vi "solar_type Script to Messages.vi"(6 "Array Delimiters (1D,2D)":string[](array[string]), 8 "error in (no error)":errorcluster, 11 "Script String":string) -> (0 "error out":errorcluster, 2 "Messages":cluster{"MSG":string, "DATA":variant}[](array[cluster]), 3 "Target":string[](array[string]), 5 "Type":enum8{"CMD", "TLM"}[](array[ring]))   [LabVIEW 2018]
doc: "This converts a SOLAR script string to one or more variant messages. Formatted as:\n<b>CMD|TLM.TARGET:PACKET{\nTYPE:VALUE,\nTYPE:'VALUE',\nTYPE|ENUM0|ENUM1|...:VALUE,\nTYPE_1D:'1,2,3',\nTYPE_2D:'1,2,3;4,5,6'}</b>\n\n<b>TYPE</b>= I8, I16, I32, I64, U8, U16, U32, U64, U8_ENUM, U16_ENUM, U32_ENUM, SGL, DBL, BOOL, STR, PATH, TIME\nTYPE_1D: 1D array (comma ',' delimited) Ex: DBL_1D:'1.23,4.567,8.92'\nTYPE_2D: 2D array (comma ',' & semicolon ';' delimited) Ex: I32_2D:'1,2,3;4,5,6'\nTYPE_ENUM: Enum with type items (pipe '|' delimited) Ex: U16_ENUM|Item 1|Item 2|Item 3:'Item 2'\n\nMyTarget:MyCMD{\nI32:-1234,\nSTR:'Hello World',\nU16_ENUM|Item1|Item2|Item3:'Item2',\nBOOL:true,\nTIME:'yyyy-mm-dd_hh:mm:ss.uuuuuu',\nPATH:'C:\\Data\\test.txt',\nU8_2D:'1,2,3;4,5,6'}"
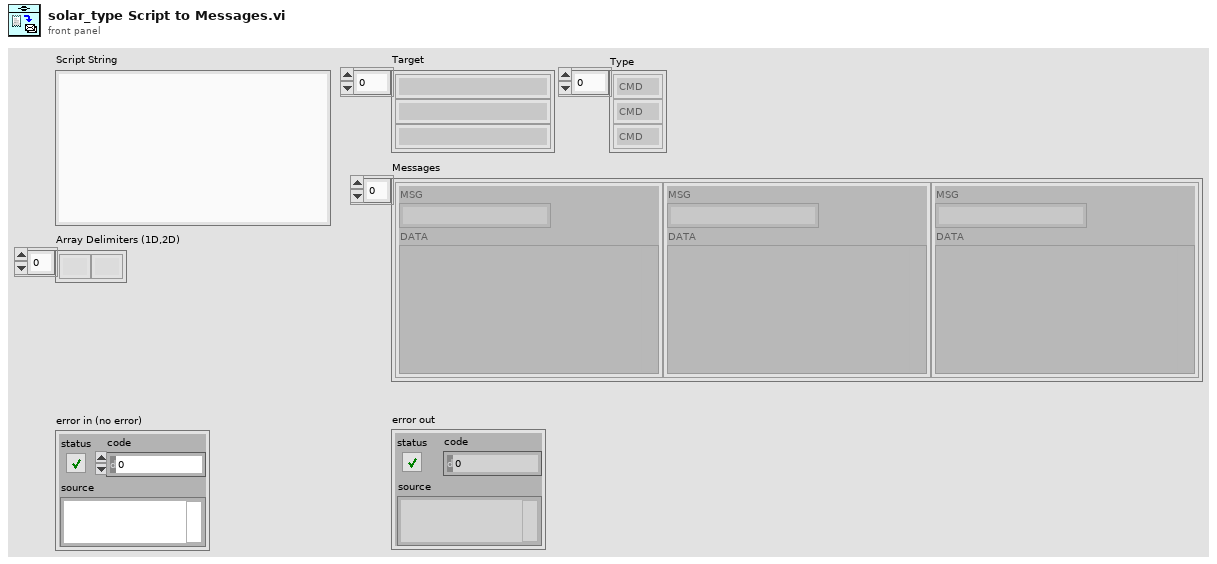
[diagram p1: front panel]
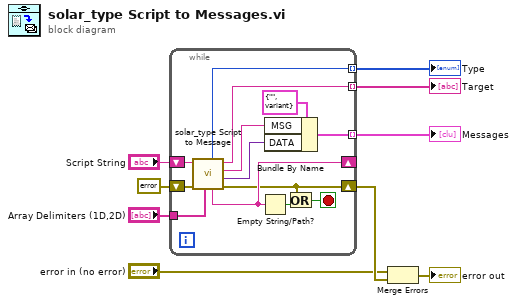
[diagram p0: block diagram]
diagram:
  n1 = while {
    shift-right: [w12] -> w8
    shift-left: errorcluster {"status"=FALSE, "code"=0, "source"=""} ("error out") -> [w22]
    shift-right: [w20] -> _
    shift-left: "Script String" -> [w21]
    tunnel: [w15] -> w3 mode=indexing
    tunnel: "Array Delimiters (1D,2D)" -> [w14]
    tunnel: [w11] -> w1 mode=indexing
    tunnel: [w10] -> w2 mode=indexing
    stop <- w13 stop-if-true
    n2 = call "solar_type Script to Message.vi"("Array Delimiters (1D,2D)"=w14, "error in (no error)"=w22, "Script String"=w21) -> ("error out"=w12:errorcluster, "Data"=w16:variant, "Packet"=w18:string, "Target"=w11:string, "Remaining"=w20:string, "Type"=w10:enum8{"CMD", "TLM"})  [unwired: 3 in]
    n3 = Empty String/Path?(string/path=w20) -> (empty?=w19:bool)
    n4 = Bundle By Name(cluster=cluster{"MSG":string, "DATA":variant} {"MSG"="", "DATA"=variant} ("Message"), "MSG"=w18, "DATA"=w16) -> (w15:cluster{"MSG":string, "DATA":variant})
    n5 = Or(x=w12, y=w19) -> (x .or. y?=w13:bool)
  }
  "Type" <- w2
  "Target" <- w1
  "Messages" <- w3
  n6 = Merge Errors("error in (no error)", w8) -> (→"error out":errorcluster)
